vi "NET GetLayerShapes.vi"(8 "error in (no error)":errorcluster, 9 "LayerId":i32, 10 "NetInputShape":i32[](array[numeric]), 11 "NET in":refnum<class "NET.lvclass">) -> (0 "error out":errorcluster, 1 "OutLayerShapes":T1[](array[typedef]), 2 "InLayerShapes":T1[](array[typedef]), 3 "NET out":refnum<class "NET.lvclass">)   [LabVIEW 2020, in "OpenLvVision_OpenCv.lvlib" / "NET.lvclass"]
doc: "Returns list of types for layer used in model."
uses:
  NET.lvclass
  C:/Users/lukas/Downloads/OpenLvVision_OpenCv/SourceCode/LabView/OpenLvVision_OpenCv/_LvHelpers/EdvrObject/EdvrObject.lvclass
  TypeDef/MatShape.ctl
  _LvHelpers/EdvrObject/EdvrObject.lvclass/EdvrObject.ctl
  OpenLvVision_OpenCv.lvlib
  _LvHelpers/EdvrObject/EdvrObject.lvclass
  Dlls/OlvOpenCvWrapper.dll
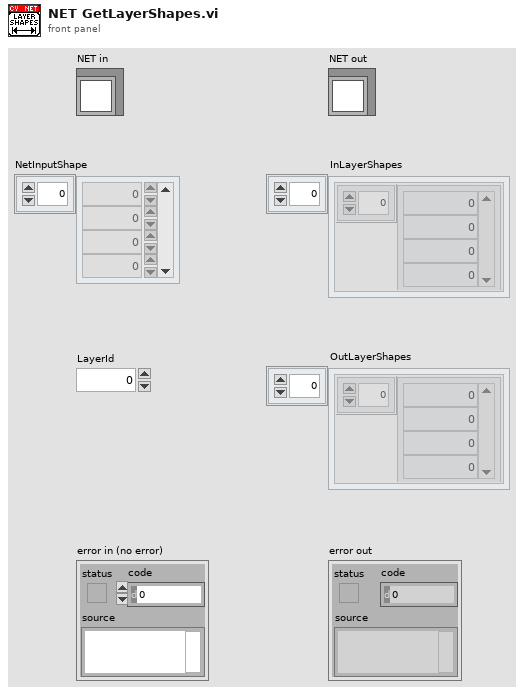
[diagram p1: front panel]
types:
  T1 = typedef "OpenLvVision_OpenCv.lvlib/MatShape.ctl" = cluster{"Data":i32[]}
  T2 = typedef "OpenLvVision_OpenCv.lvlib/EdvrObject.lvclass/Edvr.ctl" = refnum<data-value>
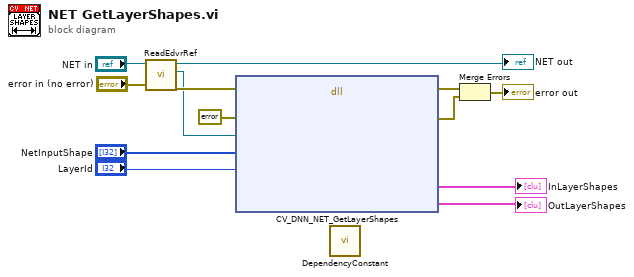
[diagram p0: block diagram]
diagram:
  n1 = call "ReadEdvrRef.vi"("error in (no error)"="error in (no error)", "EdvrObject in"="NET in") -> ("error out"=w9:errorcluster, "Edvr"=w8:T2, "EdvrObject out"=→"NET out":refnum<class "NET.lvclass">)  [unwired: 7 in]
  n2 = dll-call lib="C:/Users/lukas/Downloads/OpenLvVision_OpenCv/SourceCode/LabView/OpenLvVision_OpenCv/Dlls/OlvOpenCvWrapper.dll" fn="CV_DNN_NET_GetLayerShapes"(error in=w9, "Error"=errorcluster {"status"=FALSE, "code"=0, "source"=""} ("error out"), "edvrRef"=w8, "netInputShapeHandle"="NetInputShape", "layerId"="LayerId") -> (error out=w12:errorcluster, "Error"=w5:errorcluster, "InLayerShapes"=→"InLayerShapes":T1[], "OutLayerShapes"=→"OutLayerShapes":T1[])  [unwired: 8 in, 1 out]
  n3 = call "DependencyConstant.vi"() -> ()  [unwired: 12 in]
  n4 = Merge Errors(w12, w5) -> (→"error out":errorcluster)
